vi "LoadSetFileToDIM.vi"(1 "output array":string[][](array[string])) -> ()   [LabVIEW 2014, in "Panels.lvlib"]
uses:
  Panels.lvlib
  CS_Core/CSSystem/CoreDefs/CoreDefs.call_type.ctl
  CS_Core/BaseProcess/BaseProcess.descriptor string definition.ctl
  CS_Core/CSSystem/CoreDefs/CoreDefs.rawDataType.ctl
  CS_Core/CSSystem/CoreLib/CoreLib.short 2 byte array.vi
  CS_Core/CSSystem/CoreLib/CoreLib.double 2 byte array.vi
  CS_Core/CSSystem/CoreLib/CoreLib.string 2 byte array.vi
  CS_Core/CSSystem/CoreLib/CoreLib.lvlib
  CS_Core/BaseProcess/BaseProcess.lvlib
panel:
  in  "call cluster in":T1={"Object"="", "Selector"="", "CallType"=enum."synchronous", "Async Object"="", "Async Selector"="", "Data Descriptor"="", "Data"=[], "Error #"=0, "Expire"=0}
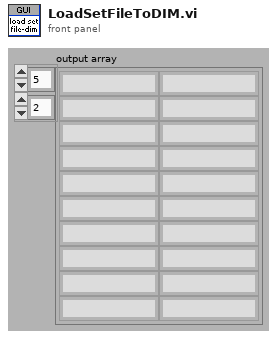
[diagram p1: front panel]
types:
  T1 = typedef "CoreDefs.call_type.ctl" = cluster{"Object":string, "Selector":string, "CallType":enum16{"simple", "synchronous", "asynchronous"}, "Async Object":string, "Async Selector":string, "Data Descriptor":T2, "Data":T3, "Error #":i32, "Expire":u32}
  T2 = typedef "BaseProcess.lvlib/BaseProcess.descriptor string definition.ctl" = string
  T3 = typedef "CoreDefs.rawDataType.ctl" = i8[]
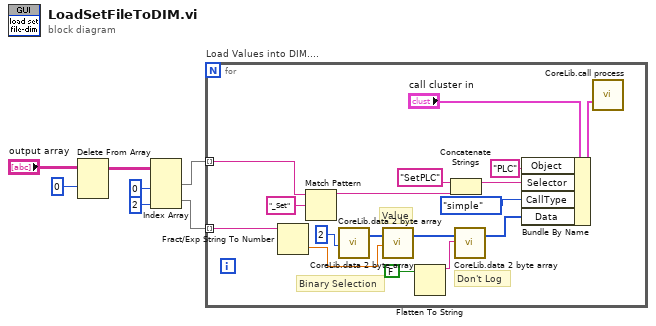
[diagram p0: block diagram]
diagram:
  n1 = Delete From Array(array="output array", index (row)=0) -> (array with subset deleted=w5:string[][])  [unwired: 2 in, 1 out]
  n2 = Index Array(array=w5, index (col) #1=0 ("disabled index (col)"), index (col) #2=2 ("index (col)")) -> (element #1=w3:string[], element #2=w2:string[])  [unwired: 2 in]
  n3 = for "Load Values into DIM...." {
    tunnel: w3 -> [w24] mode=indexing
    tunnel: w2 -> [w23] mode=indexing
    # "Don't Log"
    # "Value"
    # "Binary Selection"
    n4 = Fract/Exp String To Number(string=w23) -> (number=w8:dbl)  [unwired: 3 in, 1 out]
    n5 = Match Pattern(string=w24, regular expression="_Set") -> (before substring=w15:string)  [unwired: 1 in, 3 out]
    n6 = call-poly "CoreLib.data 2 byte array.vi"("i16"=i16 2 ("element")) -> ("byteArray out"=w10:T3)  [unwired: 18 in]
    n7 = call-poly "CoreLib.data 2 byte array.vi"("byteArray"=w10, "f64"=w8) -> ("byteArray out"=w9:T3)  [unwired: 17 in]
    n8 = Flatten To String(anything=FALSE) -> (data string=w14:string)  [unwired: 3 in, 2 out]
    n9 = Concatenate Strings("SetPLC" ("string"), w15) -> (w18:string)
    n10 = call-poly "CoreLib.data 2 byte array.vi"("byteArray"=w9, "string"=w14) -> ("byteArray out"=w13:T3)  [unwired: 17 in]
    n11 = Bundle By Name(cluster="call cluster in", "Object"="PLC", "Selector"=w18, "CallType"=enum16{"simple", "synchronous", "asynchronous"}."simple", "Data"=w13) -> (w21:T1)
    n12 = call "CoreLib.call process.vi"("call cluster in"=w21) -> ()  [unwired: 13 in, 2 out]
  }
